vi "DAQ Assistant Digital Out.vi"() -> ()   [LabVIEW 2020]
panel:
  in  "stop":bool
  in  "Digital Output":bool[](array[boolean])
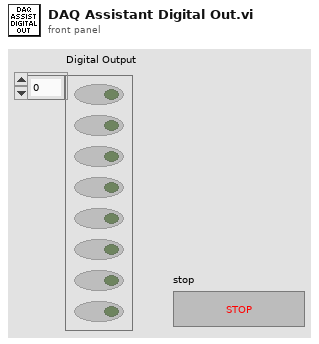
[diagram p1: front panel]
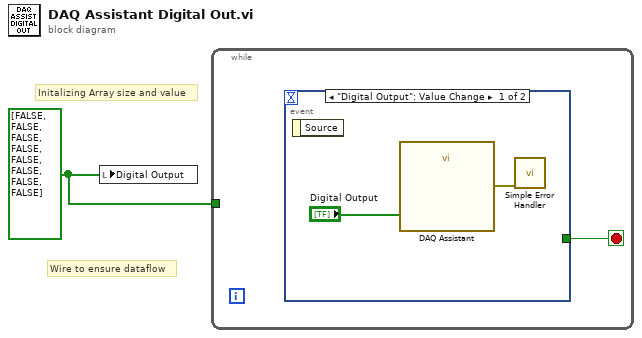
[diagram p0: block diagram]
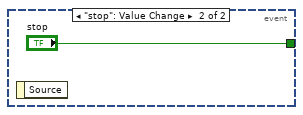
[diagram p2: hidden frame]
diagram:
  w1 = bool[] [FALSE, FALSE, FALSE, FALSE, FALSE, FALSE, FALSE, FALSE] ("Array")
  # "Initalizing Array size and value"
  # "Wire to ensure dataflow"
  n1 = local write "Digital Output"(w1) -> ()
  n2 = while {
    tunnel: w1 -> [_]
    stop <- w2 stop-if-true
    n3 = event shown="[0] \"Digital Output\": Value Change" {
      selector: _ -> [_ _]
      dyn-events: _ -> [_ _]
      timeout: _ -> [_ _]
      tunnel: [_ "stop"] -> w2
      event "Digital Output": Value Change {
        n4 = event-data() -> ()  [unwired: 1 in, 1 out]
        n5 = call "DAQ Assistant"("data"="Digital Output") -> ("error out"=w3:errorcluster)  [unwired: 17 in, 1 out]
        n6 = call <vilib>:"Simple Error Handler.vi"("error in (no error)"=w3) -> ()  [unwired: 4 in, 5 out]
      }
      event "stop": Value Change {
        n7 = event-data() -> ()  [unwired: 1 in, 1 out]
      }
    }
  }
